vi "saveGraph.vi"(8 "error in (no error)":errorcluster, 11 "dataClass in":refnum<class "SR430Class.lvclass">) -> (0 "error out":errorcluster, 3 "dataClass out":refnum<class "SR430Class.lvclass">)   [LabVIEW 2015, in "SR430Class.lvclass"]
uses:
  class/SR430Class.lvclass
  class/SR430Class.lvclass/SR430Class.ctl
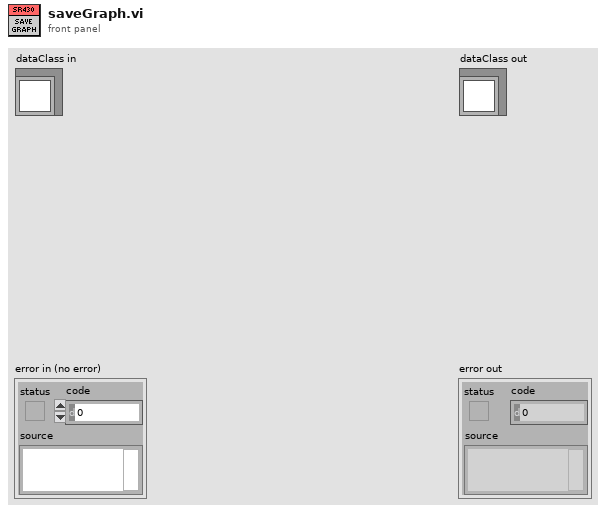
[diagram p1: front panel]
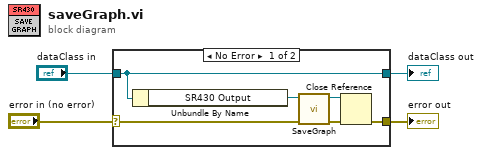
[diagram p0: block diagram]
diagram:
  n1 = case shown="No Error" "error in (no error)" {
    selector: "error in (no error)" -> [w6 w12]
    tunnel: [w5 w12] -> w3
    tunnel: [w8 w11] -> w1
    tunnel: "dataClass in" -> [w8 w11]
    frame No Error {
      n2 = Unbundle By Name(w8) -> ("SR430 Output"=w7:refnum<vi>)
      n3 = call "SaveGraph.vi"("error (in)"=w6, "reference (in)"=w7) -> ("error (out)"=w10:errorcluster, "reference (out)"=w9:refnum<vi>)  [unwired: 8 in]
      n4 = Close Reference(reference=w9, error in (no error)=w10) -> (error out=w5:errorcluster)
    }
    frame Error {
    }
  }
  "error out" <- w3
  "dataClass out" <- w1
